vi "Update a Dev Requested by UI.vi"(8 "error in (no error)":errorcluster, 10 "DevInfo":refnum<class "DevInfo.lvclass">, 11 "Controller in":refnum<class "Controller.lvclass">) -> (0 "error out":errorcluster, 3 "Controller out":refnum<class "Controller.lvclass">)   [LabVIEW 2016, in "Controller Actor.lvlib" / "Controller.lvclass"]
uses:
  <userlib>/Common Components/Controller/Controller.lvclass
  <userlib>/Common Components/Hardware/DevInfo/DevInfo.lvclass
  <userlib>/Common Components/Hardware/DevInfo/DevInfo.lvclass/DevInfo.ctl
  <userlib>/Common Components/Hardware/DevInfo/Read GUID.vi
  <userlib>/Common Components/Hardware/DevInfo/Read Device Name.vi
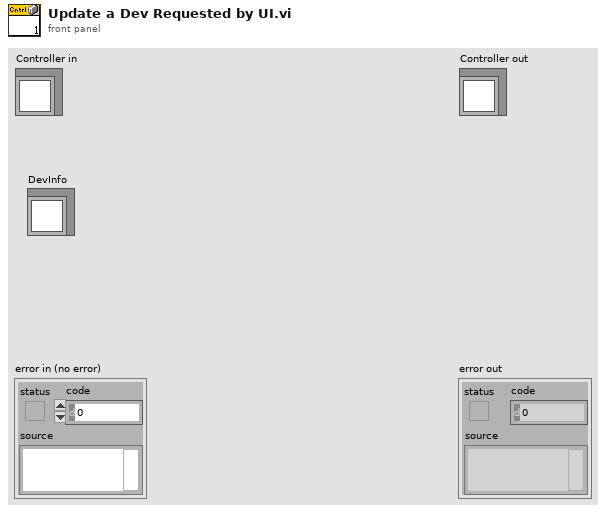
[diagram p1: front panel]
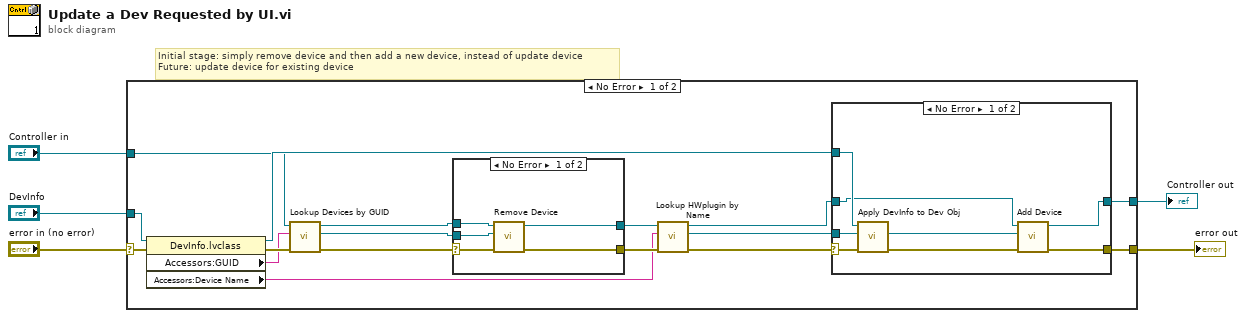
[diagram p0: block diagram]
diagram:
  # "Initial stage: simply remove device and then add a new device, instead of update device\nFuture: update device for existing device"
  n1 = case shown="No Error" "error in (no error)" {
    selector: "error in (no error)" -> [w15 w40]
    tunnel: [w18 w40] -> w4
    tunnel: "Controller in" -> [w13 w39]
    tunnel: "DevInfo" -> [w12 _]
    tunnel: [w8 w39] -> w1
    frame No Error {
      n2 = property class="DevInfo.lvclass"(reference=w12, error in=w15) -> (reference out=w22:refnum<class "DevInfo.lvclass">, error out=w14:errorcluster, "Accessors:GUID"=w6:string, "Accessors:Device Name"=w7:string)
      n3 = call <userlib>:"Lookup Devices by GUID.vi"("error in (no error)"=w14, "GUID"=w6, "Controller in"=w13) -> ("error out"=w16:errorcluster, "Dev Obj out"=w20:refnum<class "Hardware.lvclass">, "Controller out"=w19:refnum<class "Controller.lvclass">)  [unwired: 6 in]
      n4 = case shown="No Error" w16 {
        selector: w16 -> [w24 _]
        tunnel: w19 -> [w27 w28]
        tunnel: w20 -> [w23 _]
        tunnel: [w26 _] -> w11
        tunnel: [w25 w28] -> w10
        frame No Error {
          n5 = call <userlib>:"Remove Device.vi"("error in (no error)"=w24, "Device"=w23, "Controller in"=w27) -> ("error out"=w26:errorcluster, "Controller out"=w25:refnum<class "Controller.lvclass">)  [unwired: 7 in]
        }
        frame Error {
        }
      }
      n6 = call <userlib>:"Lookup HWplugin by Name.vi"("error in (no error)"=w11, "Device Name"=w7, "Controller in"=w10) -> ("error out"=w21:errorcluster, "Hardware.lvclass"=w17:refnum<class "Hardware.lvclass">, "Controller out"=w9:refnum<class "Controller.lvclass">)  [unwired: 6 in]
      n7 = case shown="No Error" w21 {
        selector: w21 -> [w34 w38]
        tunnel: w22 -> [w36 _]
        tunnel: w17 -> [w35 _]
        tunnel: [w32 w38] -> w18
        tunnel: w9 -> [w30 w37]
        tunnel: [w31 w37] -> w8
        frame No Error {
          n8 = call <userlib>:"Apply DevInfo to Dev Obj.vi"("error in (no error)"=w34, "Dev Obj in"=w35, "DevInfo in"=w36) -> ("error out"=w33:errorcluster, "Dev Obj out"=w29:refnum<class "Hardware.lvclass">)  [unwired: 6 in, 1 out]
          n9 = call <userlib>:"Add Device.vi"("error in (no error)"=w33, "Device"=w29, "Controller in"=w30) -> ("error out"=w32:errorcluster, "Controller out"=w31:refnum<class "Controller.lvclass">)  [unwired: 7 in]
        }
        frame Error {
        }
      }
    }
    frame Error {
    }
  }
  "error out" <- w4
  "Controller out" <- w1
